vi "Dashboard Main.vi"() -> ()   [LabVIEW 2015]
uses:
  <vilib>/event_ctls.llb/eventvkey.ctl
  <vilib>/Utility/config.llb/NI_LVConfig.lvlib
  <vilib>/Utility/config.llb/Write Key (I32).vi
  <vilib>/Rock Robotics/WPI/Dashboard/WPI_DashboardLogging Global.vi
  <vilib>/Utility/config.llb/Write Key (String).vi
  <vilib>/Rock Robotics/Network Tables/NT Read Numeric Array.vi
  <vilib>/Utility/miscctls.llb/LVRowAndColumnTypeDef.ctl
panel:
  in  "TCP":refnum<k5>
  in  "Rec Mode":enum32{"Stop", "Record", "Playback"}(radio)
  in  "Vision":u16(ring) items=["Camera Off", "USB Camera SW", "USB Camera HW", "IP Camera"]
  out "Camera IP":string
  out "Image Message":string="Timeout in Camera Communications"
  in  "Dashboard Tab":T1(tab)
  in  "Select Auto":string(combo)
  out "NT Connection":bool
  in  "Camera Settings":T2={"Frame Rate"=30, "Compression"=30, "Size"=1} {"Frame Rate" scale=1.0..30.0; "Size" items=["640x480", "320x240", "160x120"]}
  out "MotorChart R":cluster{"Numeric":dbl, "Numeric":dbl}(graph)
  out "MotorChart L":T3(graph)
  out "MotorSliders R":cluster{"MotorSlide1":dbl, "MotorSlide2":dbl} {"MotorSlide2" scale=-1.0..1.0 scale format="%#_2e"; "MotorSlide1" scale=-1.0..1.0 scale format="%#_2e"}
  out "MotorSliders L":T4 {"MotorSlide4 2" scale=0.0..14.0 scale format="%#_2e"; "MotorSlide2" scale=-1.0..1.0 scale format="%#_2e"; "MotorSlide1" scale=-1.0..1.0 scale format="%#_2e"}
  out "Gyro":dbl(knob) scale=0.0..360.0
  out "JS1 Z":dbl(slide) scale=-1.0..1.0 scale format="%#_2e"
  out "JS1 Graph":cluster{"X":dbl, "Y":dbl}[](graph)
  out "JS1 Buttons":T5
  out "JS2 Z":dbl(slide) scale=-1.0..1.0 scale format="%#_2e"
  out "JS2 Graph":cluster{"X":dbl, "Y":dbl}[](graph)
  out "JS2 Buttons":T5
  out "Mode":T6(ring)=enum."Auto Disabled"
  in  "DB Camera Config":bool
  out "fps":dbl format="%#.1g"
  out "Mbps":dbl format="%#.1g"
  out "Mbps LED":bool
  in  "DB/String 9":string
  in  "DB/String 8":string
  in  "DB/String 7":string
  in  "DB/String 6":string
  in  "DB/String 5":string
  in  "DB/String 4":string
  in  "DB/String 3":string
  in  "DB/String 2":string
  in  "DB/String 1":string
  in  "DB/String 0":string
  in  "DB/Slider 0":dbl(slide) scale=0.0..5.0
  in  "DB/Slider 1":dbl(slide) scale=0.0..5.0
  in  "DB/Slider 2":dbl(slide) scale=0.0..5.0
  in  "DB/Slider 3":dbl(slide) scale=0.0..5.0
  out "DB/LED 3":bool
  out "DB/LED 2":bool
  out "DB/LED 1":bool
  out "DB/LED 0":bool
  in  "DB/Button 3":bool
  in  "DB/Button 2":bool
  in  "DB/Button 1":bool
  in  "DB/Button 0":bool caption="New Name"
  out "Aim":bool
  out "Shooter":bool
  out "Drive":bool
  in  "Strategty":i8 min=0 max=4
  in  "Test Slider":dbl(slide) scale=0.0..100.0 scale format="%#_3g"
  in  "On/Off":bool caption="Solenoid"
  in  "Test Name":u16(ring) items=["Select the test to run..."]
  in  "Test Tree":string(tree)
  in  "Motor":cluster{"Value":dbl, "Enable":bool} {"Value" scale=-1.0..1.0 scale format="%#_3g"}
  out "Progress":T7 {"Test Progress" scale=0.0..100.0}
  in  "Rev/Fwd":cluster{"Forward":bool, "Reverse":bool}
  in  "Test Ring":u16(ring) items=["Monochrome", "Color"]
  out "Cmd Status":string
  in  "Execute Command":bool
  in  "Command Params":string[][](table)
  in  "Command Selection":i32(listbox)
  in  "CheckList":i32(listbox)
  out "Tree":string(tree)
  out "Camera Image":T8(plugin-control)
  # "Left"
  # "Front"
  # "Right"
  # "Battery"
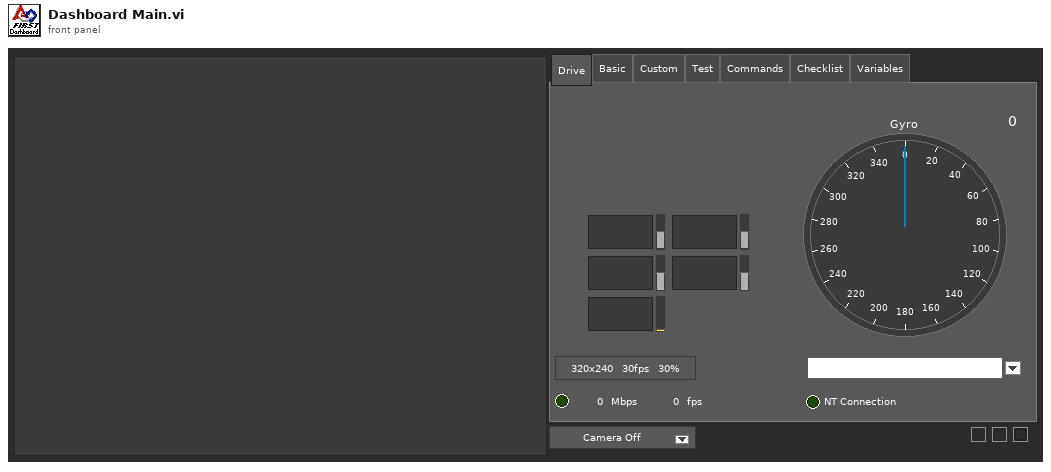
[diagram p1: front panel]
types:
  T1 = enum32{"Drive", "Basic", "Custom", "Test", "Commands", "Checklist", "Variables"}
  T2 = cluster{"Frame Rate":i32, "Compression":i32, "Size":u16}
  T3 = cluster{"Numeric":dbl, "Numeric":dbl, "Battery V":dbl}
  T4 = cluster{"MotorSlide1":dbl, "MotorSlide2":dbl, "MotorSlide4 2":dbl}
  T5 = cluster{bool, bool, bool, bool, bool, bool, bool, bool, bool, bool, bool, bool}
  T6 = enum8{"Tele-Op Disabled", "Tele-Op Enabled", "Auto Disabled", "Auto Enabled", "Test Disabled", "Test Enabled", "Disconnected", "No Code", "E-Stop"}
  T7 = cluster{"Test Progress":u8, "Test Progress Text":string}
  T8 = typedef "IMAQ Image.ctl" = refnum<image>
  T9 = cluster{"IDs":cluster{"RPC field ID":u16, "Unique ID":u16}, "String":string}
  T10 = enum32{"Drive", "Basic", "Custom", "Test", "Checklist", "Variables"}
  T11 = typedef "Image Type" = u32
  T12 = cluster{"Camera Image":refnum<vi>, "Dashboard Tab":refnum<vi>, void, "Vision":refnum<vi>, "Rec Mode":refnum<vi>, "Test Slider":refnum<vi>, "On/Off ":refnum<vi>, "Test Ring":refnum<vi>, "Rev/Fwd":refnum<vi>, "Test Name":refnum<vi>, "Motor":refnum<vi>, "Progress":refnum<vi>, "CheckList":refnum<vi>, "Tree":refnum<vi>, "Test Tree":refnum<vi>, "Command Params":refnum<vi>, "Command Selection":refnum<vi>, "Execute Command":refnum<vi>, "Cmd Status":refnum<vi>}
  T13 = cluster{"Error Strings":string, "Disable Counts":cluster{u16, u16}, "Rail Faults":cluster{u16, u16, u16}, "Robot IP":string, "DB Mode":u8, "Event Info":cluster{"Name":string, "Type":u8, "Number":u16, "Replay":u8}, "Camera Addr":string}
  T14 = cluster{"Storage":cluster{"Disk Free":u64, "RAM Block":u32, "RAM free":u32}, "CPU Utilization":cluster{"CPU % ISR":sgl, "CPU % Time Crit":sgl, "CPU % Timed Str":sgl, "CPU % High":sgl, "CPU % Above":sgl, "CPU % Normal":sgl, "CPU % Low":sgl}, "CAN":cluster{"% Bus Utilization":sgl, "Bus Off Cnt":u32, "TX_FIFO Full Cnt":u32, "Receive Error Cnt":u8, "Transmit Error Cnt":u8}, "HID":cluster{"HID Outputs":u32, "Rumble Low":u16, "Rumble High":u16}[]}
  T15 = cluster{"Status bits":cluster{"Test Mode":bool, "Autonomous":bool, "Enabled":bool, "Code Start":bool, "Brownout":bool, "Reserved 2":bool, "Reserved 3":bool, "E-Stop":bool}, "Code Trace":cluster{"Disabled":bool, "TeleOp":bool, "Auto":bool, "Test":bool}, "Controller Type":enum16{"unknown", "cRIO", "roboRio"}, "Code?":enum16{"unknown", "noCode", "code"}, "Battery V":dbl}
  T16 = cluster{"Control Bits":cluster{"TestMode":bool, "Autonomous":bool, "Enabled":bool, "FMS Present":bool, bool, bool, bool, "E-Stop":bool}, "Team Station ":u8, "Countdown":sgl, "Joystick Values":cluster{"Axes":dbl[], "Buttons":bool[], "POVs":i16[]}[]}
  T17 = cluster{"Axes":dbl[], "Buttons":bool[], "POVs":i16[]}[]
  T18 = cluster{"Axes":dbl[], "Buttons":bool[], "POVs":i16[]}
  T19 = cluster{"Buttons[0]":bool, "Buttons[1]":bool, "Buttons[2]":bool, "Buttons[3]":bool, "Buttons[4]":bool, "Buttons[5]":bool, "Buttons[6]":bool, "Buttons[7]":bool, "Buttons[8]":bool, "Buttons[9]":bool, "Buttons[10]":bool, "Buttons[11]":bool}
  T20 = typedef "NI_LVConfig.lvlib/Config Data RefNum.ctl" = refnum<k1>
  T21 = cluster{"Operation":enum16{"Update", "Clear"}, "Color Box":u32}[]
  T22 = typedef "eventvkey.ctl" = enum16{"ASCII", "Enter", "Return", "Shift", "Ctrl", "Alt", "Cmd", "Opt", "Caps", "NumLock", "Clear", "Break", "Up", "Down", "Left", "Right", "Insert", "Delete", "Home", "End", "PageUp", "PageDown", "Escape", "Help", "Pause", "ScrollLock", "F1", "F2", "F3", "F4", "F5", "F6", "F7", "F8", "F9", "F10", "F11", "F12", "F13", "F14", "F15", "F16", "F17", "F18", "F19", "F20", "F21", "F22", "F23", "F24", "Play", "VolumeUp", "VolumeDown", "Mute", "Two Byte Char"}
  T23 = cluster{"Image Size":bool, "Image Type":bool, "Pixel Value":bool, "ROI Information":bool, "Zoom Factor":bool}
  T24 = enum8{"Enabled", "Disabled", "Disabled and Grayed Out"}
  T25 = cluster{"Operation":enum16{"Update", "Clear"}, "Color Box":u32}
  T26 = typedef "LVRowAndColumnTypeDef.ctl" = cluster{"Row":i32, "Column":i32}
  T27 = cluster{"Shift":bool, "Ctrl":bool, "Alt":bool, "Cmd":bool, "Opt":bool}
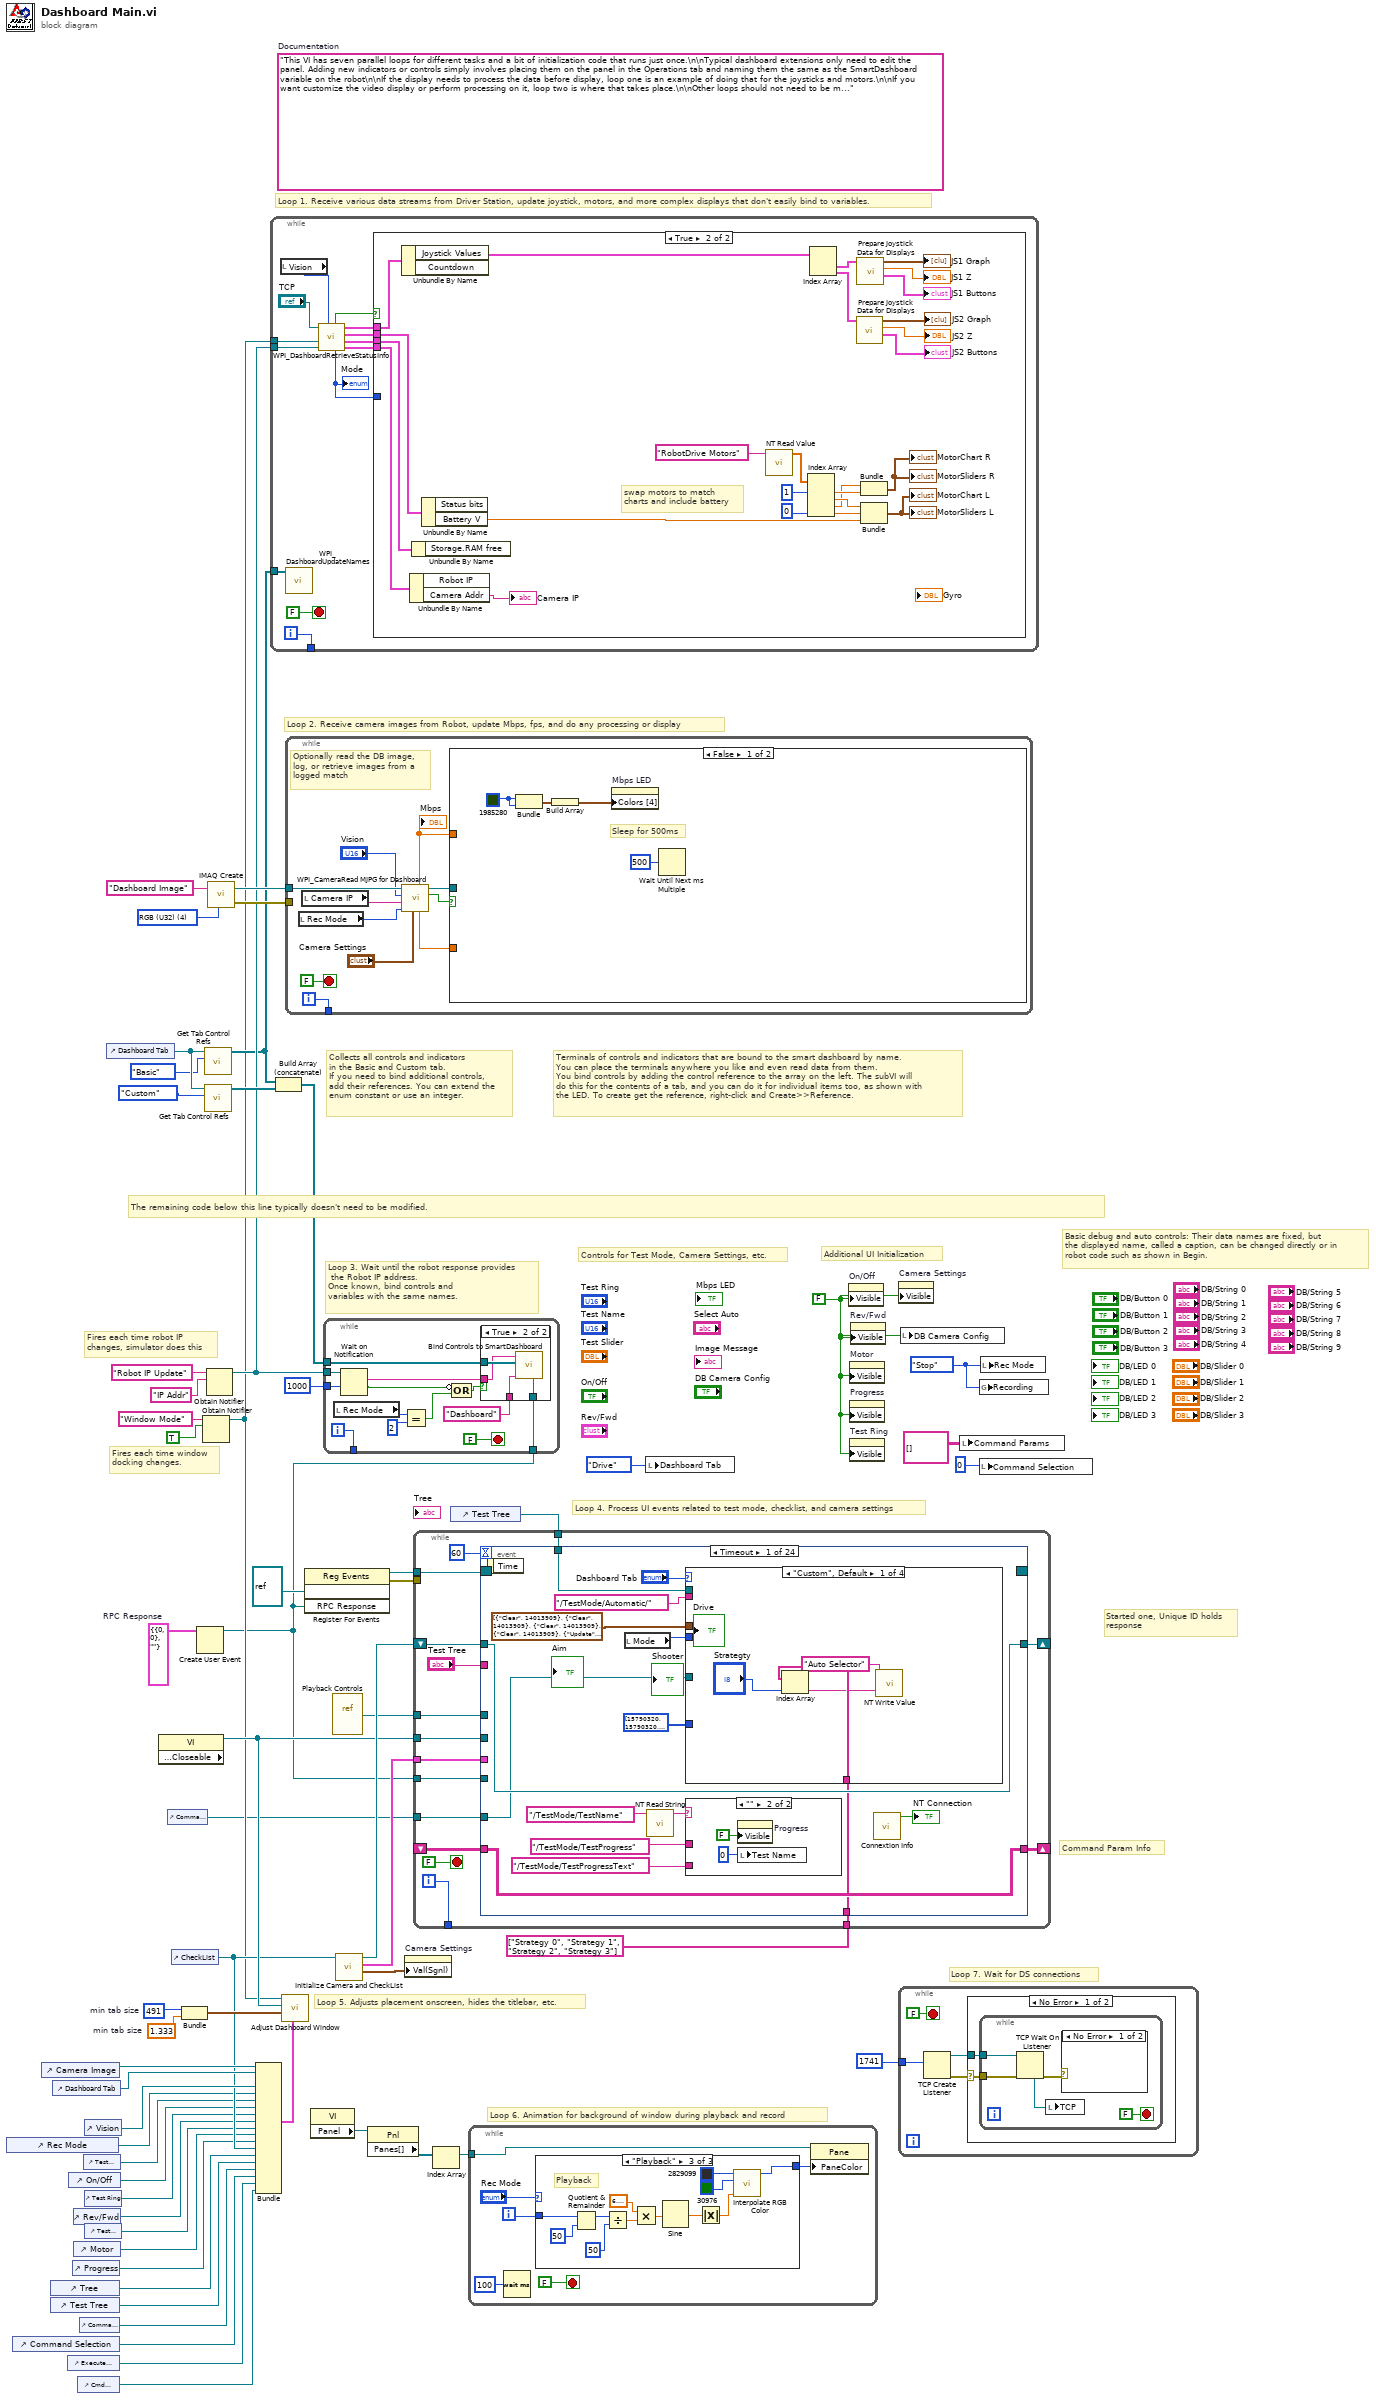
[diagram p0: block diagram]
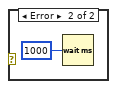
[diagram p2: hidden frame]
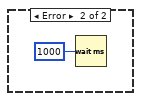
[diagram p3: hidden frame]
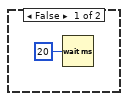
[diagram p4: hidden frame]
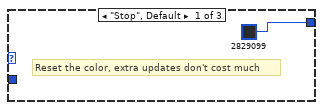
[diagram p5: hidden frame]
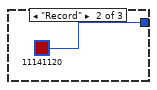
[diagram p6: hidden frame]
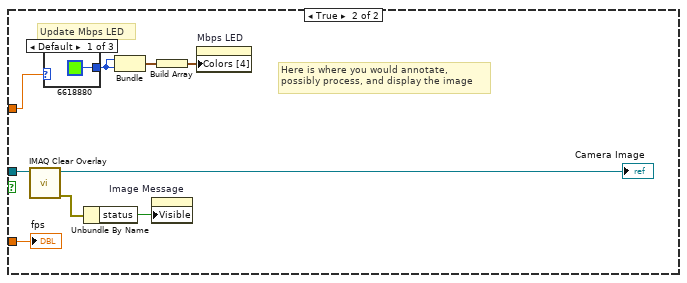
[diagram p8: hidden frame]
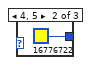
[diagram p9: hidden frame]
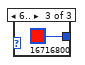
[diagram p10: hidden frame]
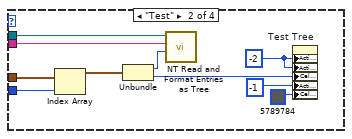
[diagram p11: hidden frame]
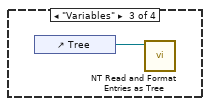
[diagram p12: hidden frame]
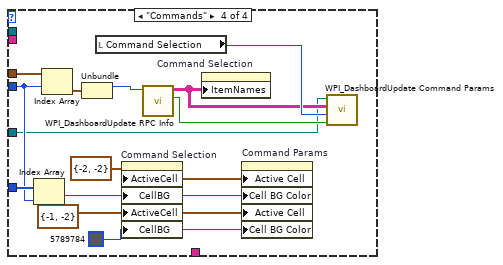
[diagram p13: hidden frame]
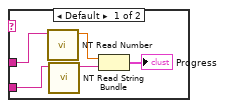
[diagram p14: hidden frame]
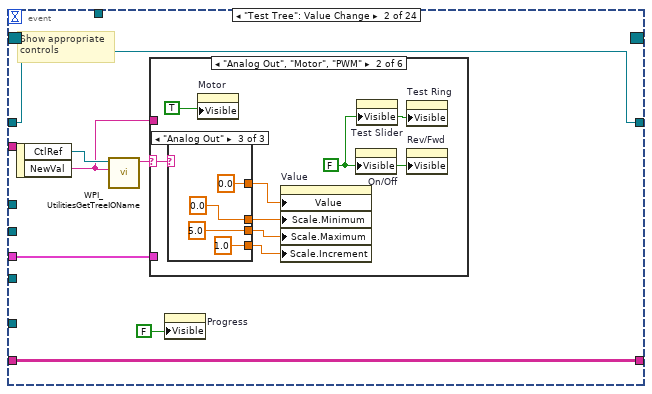
[diagram p15: hidden frame]
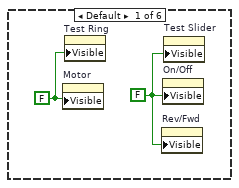
[diagram p16: hidden frame]
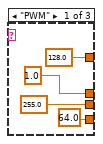
[diagram p17: hidden frame]
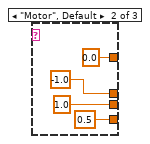
[diagram p18: hidden frame]
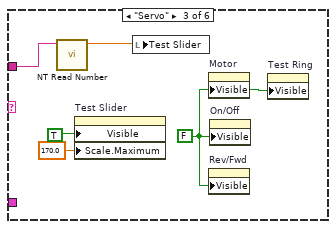
[diagram p19: hidden frame]
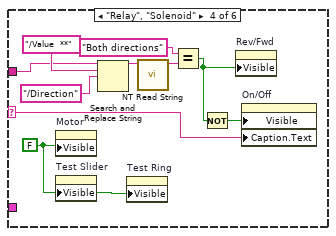
[diagram p20: hidden frame]
diagram:
  w8 = T9 {"IDs"={"RPC field ID"=0, "Unique ID"=0}, "String"=""}  # RPC Response
  w34 = 491  # min tab size
  w33 = 1.333  # min tab size
  w42 = enum32{"Stop", "Record", "Playback"}."Stop" ("Rec Mode")
  w16 = FALSE ("Visible")
  (unwired) "This VI has seven parallel loops for different tasks and a bit of initialization code that runs just once.\n\nTypical dashboard extensions only need to edit the panel. Adding new indicators or controls simply involves placing them on the panel in the Operations tab and naming them the same as the SmartDashboard variable on the robot\n\nIf the display needs to process the data before display, loop one is an example of doing that for the joysticks and motors.\n\nIf you want customize the video display or perform processing on it, loop two is where that takes place.\n\nOther loops should not need to be modified. They are pretty standard, and document the task they perform."  # Documentation
  w62 = T11 4 items=["Grayscale (U8)", "Grayscale (I16)", "Grayscale (SGL)", "Complex (CSG)", "RGB (U32)", "HSL (U32)", "RGB (U64)"] ("Image Type")
  # "Command Param Info"
  # "Started one, Unique ID holds\nresponse"
  # "Loop 7. Wait for DS connections"
  # "Basic debug and auto controls: Their data names are fixed, but\nthe displayed name, called a caption, can be changed directly or in\nrobot code such as shown in Begin."
  # "Controls for Test Mode, Camera Settings, etc."
  # "Additional UI Initialization"
  # "Loop 6. Animation for background of window during playback and record"
  # "Fires each time robot IP\nchanges, simulator does this"
  # "Fires each time window\ndocking changes."
  # "Collects all controls and indicators\nin the Basic and Custom tab.\nIf you need to bind additional controls,\nadd their references. You can extend the\nenum constant or use an integer."
  # "The remaining code below this line typically doesn't need to be modified."
  # "Loop 4. Process UI events related to test mode, checklist, and camera settings"
  # "Terminals of controls and indicators that are bound to the smart dashboard by name.\nYou can place the terminals anywhere you like and even read data from them.\nYou bind controls by adding the control reference to the array on the left. The subVI will\ndo this for the contents of a tab, and you can do it for individual items too, as shown with\nthe LED. To create get the reference, right-click and Create>>Reference."
  # "Loop 3. Wait until the robot response provides\n the Robot IP address.\nOnce known, bind controls and\nvariables with the same names."
  # "Loop 5. Adjusts placement onscreen, hides the titlebar, etc."
  # "Loop 1. Receive various data streams from Driver Station, update joystick, motors, and more complex displays that don't easily bind to variables."
  # "Loop 2. Receive camera images from Robot, update Mbps, fps, and do any processing or display"
  n1 = control-ref of="Rec Mode"() -> (w22:refnum<vi>)
  n2 = control-ref of="Command Selection"() -> (w7:refnum<vi>)
  n3 = control-ref of="Camera Image"() -> (w37:refnum<vi>)
  n4 = control-ref of="Tree"() -> (w26:refnum<vi>)
  n5 = control-ref of="Test Tree"() -> (w25:refnum<vi>)
  n6 = control-ref of="Dashboard Tab"() -> (w36:refnum<vi>)
  n7 = control-ref of="Execute Command"() -> (w9:refnum<vi>)
  n8 = control-ref of="On/Off"() -> (w20:refnum<vi>)
  n9 = control-ref of="Progress"() -> (w17:refnum<vi>)
  n10 = control-ref of="Rev/Fwd"() -> (w18:refnum<vi>)
  n11 = control-ref of="Motor"() -> (w23:refnum<vi>)
  n12 = control-ref of="Cmd Status"() -> (w3:refnum<vi>)
  n13 = control-ref of="Command Params"() -> (w10:refnum<vi>)
  n14 = control-ref of="Test Slider"() -> (w21:refnum<vi>)
  n15 = control-ref of="Vision"() -> (w35:refnum<vi>)
  n16 = control-ref of="Test Ring"() -> (w19:refnum<vi>)
  n17 = control-ref of="Test Name"() -> (w24:refnum<vi>)
  n18 = control-ref of="Dashboard Tab"() -> (w40:refnum<vi>)
  n19 = property class="VI" props=["Front Panel.Closeable"]() -> (reference out=w41:refnum<vi>)  [unwired: 2 in, 2 out]
  n20 = control-ref of="Command Params"() -> (w2:refnum<vi>)
  n21 = control-ref of="CheckList"() -> (w27:refnum<vi>)
  n22 = Bundle("min tab size"=w34, "min tab size"=w33) -> (w32:cluster{"min tab size":i32, "min tab size":dbl})  [unwired: 1 in]
  n23 = Create User Event(user event datatype=w8) -> (user event=w4:refnum<user-event>)  [unwired: 1 in, 1 out]
  n24 = Obtain Notifier(name (unnamed)="Window Mode", notification data type=TRUE) -> (notifier out=w13:refnum<notifier>)  [unwired: 2 in, 2 out]
  n25 = call <vilib>:"Get Tab Control Refs.vi"("Page Index"=T10."Basic" ("Dashboard Tab"), "TabControl in"=w40) -> ("ControlsOnPage"=w14:refnum<vi>[])  [unwired: 9 in]
  n26 = call <vilib>:"Get Tab Control Refs.vi"("Page Index"=T10."Custom" ("Dashboard Tab"), "TabControl in"=w40) -> ("ControlsOnPage"=w39:refnum<vi>[])  [unwired: 9 in]
  n27 = Obtain Notifier(name (unnamed)="Robot IP Update", notification data type="IP Addr" ("name (unnamed)")) -> (notifier out=w15:refnum<notifier>)  [unwired: 2 in, 2 out]
  n28 = call "IMAQ Create"("Image Name"="Dashboard Image", "Image Type"=w62) -> ("New Image"=w60:T8, "error out"=w59:errorcluster)  [unwired: 2 in, 1 out]
  n29 = Bundle("Camera Image"=w37, "Dashboard Tab"=w36, "Vision"=w35, "Rec Mode"=w22, "Test Slider"=w21, "On/Off"=w20, "Test Ring"=w19, "Rev/Fwd"=w18, "Test Name"=w24, "Motor"=w23, "Progress"=w17, "CheckList"=w27, "Tree"=w26, "Test Tree"=w25, "Command Params"=w10, "Command Selection"=w7, "Execute Command"=w9, "Cmd Status"=w3) -> (w28:T12, w31)  [unwired: 1 in]
  n30 = while {
    tunnel: [w74] -> _
    tunnel: w15 -> [w68]
    tunnel: w14 -> [w67]
    tunnel: w13 -> [w63]
    i -> [w74]
    stop <- FALSE stop-if-true
    n31 = local read "Vision"() -> (w65:u16)
    n32 = call <vilib>:"WPI_DashboardUpdateNames.vi"("Controls on Tab"=w67) -> ()  [unwired: 11 in]
    n33 = call <vilib>:"WPI_DashboardRetrieveStatusInfo.vi"("Vision"=w65, "Binding Refnum"=w68, "Window Mode Notifier"=w63, "TCP Cnx"="TCP") -> ("Power and Errors"=w69:T13, "Robot Metrics"=w72:T14, "Status Info"=w73:T15, "Control Info"=w70:T16, "Robot Mode"=w66:T6, "Process?"=w71:bool)  [unwired: 2 in]
    "Mode" <- w66
    n34 = case shown="True" w71 {
      tunnel: w73 -> [_ w101]
      tunnel: w72 -> [_ w100]
      tunnel: w70 -> [_ w99]
      tunnel: w69 -> [_ w98]
      tunnel: w66 -> [_ _]
      frame False {
        n35 = Wait (ms)(milliseconds to wait=u32 20) -> ()  [unwired: 1 out]
      }
      frame True {
        # "swap motors to match\ncharts and include battery"
        n36 = Unbundle By Name(w99) -> ("Joystick Values"=w88:T17)  [unwired: 1 out]
        n37 = Unbundle By Name(w98) -> ("Camera Addr"=→"Camera IP":string)  [unwired: 1 out]
        n38 = Unbundle By Name(w100) -> ()  [unwired: 1 out]
        n39 = Unbundle By Name(w101) -> ("Battery V"=w89:dbl)  [unwired: 1 out]
        n40 = call-poly <vilib>:"NT Read Value.vi"("Name"="RobotDrive Motors") -> ("Numeric Array"=w77:dbl[])  [unwired: 9 in, 1 out]
        n41 = Index Array(array=w77, index #1=1, index #4=0) -> (element #1=w93:dbl, element #2=w94:dbl, element #3=w92:dbl, element #4=w97:dbl)  [unwired: 2 in]
        n42 = Index Array(array=w88) -> (element #1=w87:T18, element #2=w82:T18)  [unwired: 2 in]
        n43 = call "Prepare Joystick Data for Displays.vi"("Joystick Values"=w82) -> ("Buttons"=→"JS2 Buttons":T19, "Z Axis"=→"JS2 Z":dbl, "Cartesian Data"=→"JS2 Graph":cluster{"X axis":dbl, "X axis":dbl}[])  [unwired: 8 in]
        n44 = call "Prepare Joystick Data for Displays.vi"("Joystick Values"=w87) -> ("Buttons"=→"JS1 Buttons":T19, "Z Axis"=→"JS1 Z":dbl, "Cartesian Data"=→"JS1 Graph":cluster{"X axis":dbl, "X axis":dbl}[])  [unwired: 8 in]
        n45 = Bundle("Numeric"=w92, "Numeric"=w93) -> (→"MotorChart R" →"MotorSliders R":cluster{"Numeric":dbl, "Numeric":dbl})  [unwired: 1 in]
        n46 = Bundle("Numeric"=w94, "Numeric"=w97, "Battery V"=w89) -> (→"MotorChart L" →"MotorSliders L":T3)  [unwired: 1 in]
      }
    }
  }
  n47 = Build Array (concatenate)(w14, w39) -> (w38:refnum<vi>[])
  n48 = call "Adjust Dashboard Window.vi"("Sizing Refnums"=w28, "Size Constraints"=w32, "VI"=w41, "WIn Mode"=w13) -> ()  [unwired: 8 in]
  n49 = while {
    tunnel: w60 -> [w110]
    tunnel: w59 -> [_]
    tunnel: [w111] -> _
    i -> [w111]
    stop <- FALSE stop-if-true
    # "Optionally read the DB image,\nlog, or retrieve images from a\nlogged match"
    n50 = local read "Rec Mode"() -> (w105:enum32{"Stop", "Record", "Playback"})
    n51 = local read "Camera IP"() -> (w103:string)
    n52 = call <vilib>:"WPI_CameraRead MJPG for Dashboard.vi"("Camera Settings"="Camera Settings", "Rec Mode"=w105, "Camera IP"=w103, "Camera Mode"="Vision", "Refnum in"=w110) -> ("Active"=w108:bool, "Refnum out"=w109:T8, "FPS"=w107:dbl, "Bandwidth (Mbps)"=w102:dbl)  [unwired: 3 in]
    "Mbps" <- w102
    n53 = case shown="False" w108 {
      tunnel: w109 -> [_ w120]
      tunnel: w102 -> [_ w119]
      tunnel: w107 -> [_ w117]
      frame False {
        w113 = u32 1985280 ("Color Box")
        # "Sleep for 500ms"
        n54 = Bundle("Color Box"=w113, "Color Box"=w113) -> (w115:cluster{"Color Box":u32, "Color Box":u32})  [unwired: 1 out]
        n55 = Build Array(w115) -> (w114:cluster{"Color Box":u32, "Color Box":u32}[])
        n56 = property on="Mbps LED" class="Bool (strict)"("Colors [4]"=w114) -> ()  [unwired: 2 in, 2 out]
        n57 = Wait Until Next ms Multiple(millisecond multiple=u32 500) -> ()  [unwired: 1 out]
      }
      frame True {
        # "Here is where you would annotate,\npossibly process, and display the image"
        # "Update Mbps LED"
        n58 = call "IMAQ Clear Overlay"("Image"=w120) -> ("error out"=w124:errorcluster, "Image Out"=→"Camera Image":T8)  [unwired: 2 in, 7 out]
        n59 = case shown="Default" w119 {
          tunnel: [u32 6618880 ("Color Box") u32 16776722 ("Color Box") u32 16716800 ("Color Box")] -> w121
          frame Default {
          }
          frame 4, 5 {
          }
          frame 6.. {
          }
        }
        n60 = Unbundle By Name(w124) -> ("status"=w125:bool)
        n61 = Bundle("Color Box"=w121, "Color Box"=w121) -> (w123:cluster{"Color Box":u32, "Color Box":u32})  [unwired: 1 out]
        n62 = property on="Image Message" class="Str"("Visible"=w125) -> ()  [unwired: 2 in, 2 out]
        n63 = Build Array(w123) -> (w122:cluster{"Color Box":u32, "Color Box":u32}[])
        n64 = property on="Mbps LED" class="Bool (strict)"("Colors [4]"=w122) -> ()  [unwired: 2 in, 2 out]
        "fps" <- w117
      }
    }
  }
  n65 = register-events(refnum<vi> refnum, w4) -> (reference out=w46:refnum<event-registration>, error out=w45:errorcluster)  [unwired: 2 in]
  n66 = property class="VI"() -> ("Panel"=w49:refnum<vi>)  [unwired: 2 in, 2 out]
  n67 = while {
    tunnel: w38 -> [w141]
    tunnel: w15 -> [w139]
    tunnel: [w137] -> _
    tunnel: u32 1000 ("milliseconds to wait") -> [w136]
    tunnel: w4 -> [w129]
    i -> [w137]
    stop <- FALSE stop-if-true
    n68 = local read "Rec Mode"() -> (w132:enum32{"Stop", "Record", "Playback"})
    n69 = Wait on Notification(notifier=w139, timeout in ms (-1)=w136) -> (notification=w138:string, timed out?=w134:bool)  [unwired: 2 in, 2 out]
    n70 = Equal?(x=w132, y=u16 2 ("Rec Mode")) -> (x = y?=w133:bool)
    n71 = Compound Arithmetic op=OR(invert w134, w133) -> (w135:bool)
    n72 = case shown="True" w135 {
      tunnel: w141 -> [_ w145]
      tunnel: w138 -> [_ w144]
      tunnel: "Dashboard" -> [_ w143]
      tunnel: w129 -> [_ w142]
      frame False {
      }
      frame True {
        n73 = call <vilib>:"Bind Controls to SmartDashboard.vi"("RPC ref"=w142, "Client Name"=w143, "Bound Control Refs"=w145, "Server IP Address"=w144) -> ()  [unwired: 8 in]
      }
    }
  }
  n74 = vi-ref "Playback Controls.vi"() -> (w47:refnum<vi>)
  n75 = call "Initialize Camera and CheckList.vi"("ListBox in"=w27) -> ("Cluster"=w53:cluster{"value":i32, "value":i32, "index":i32}, "Array"=w54:cluster{string[]}[], "File Refnum"=w52:T20)  [unwired: 8 in]
  n76 = property class="Pnl"(reference=w49) -> ("Panes[]"=w50:refnum<vi>[])  [unwired: 1 in, 2 out]
  n77 = property on="Camera Settings" class="Clust (strict)"("Val(Sgnl)"=w53) -> ()  [unwired: 2 in, 2 out]
  n78 = Index Array(array=w50) -> (element=w48:refnum<vi>)  [unwired: 1 in]
  n79 = control-ref of="Test Tree"() -> (w51:refnum<vi>)
  n80 = while {
    tunnel: w54 -> [w158]
    shift-right: [w157] -> _
    shift-left: w52 -> [w156]
    tunnel: [w155] -> _
    tunnel: w51 -> [w154]
    tunnel: w47 -> [w153]
    tunnel: w46 -> [w152]
    tunnel: w45 -> [_]
    tunnel: w41 -> [w151]
    tunnel: w4 -> [w150]
    tunnel: w2 -> [w149]
    shift-right: [w148] -> _
    shift-left: _ -> [w147]
    tunnel: string[] ["Strategy 0", "Strategy 1", "Strategy 2", "Strategy 3"] -> [w146]
    i -> [w155]
    stop <- FALSE stop-if-true
    n81 = event shown="[0] Timeout" {
      selector: w152 -> [_ _ _ _ _ _ _ _ _ _ _ _ _ _ _ _ _ _ _ _ _ _ _ _]
      dyn-events: [_ _ _ _ _ _ _ _ _ _ _ _ _ _ _ _ _ _ w472 _ _ _ _ _] -> _
      timeout: u32 60 ("milliseconds to wait") -> [_ _ _ _ _ _ _ _ _ _ _ _ _ _ _ _ _ _ _ _ _ _ _ _]
      tunnel: w154 -> [w172 _ _ _ _ _ _ _ _ _ _ _ _ _ _ _ _ _ _ _ _ _ _ _]
      tunnel: "Test Tree" -> [_ _ _ _ _ _ _ _ _ _ _ _ _ w435 w444 w447 w452 w461 _ _ _ _ _ _]
      tunnel: w158 -> [_ w214 _ _ _ _ _ _ _ _ _ w397 w428 _ _ _ _ _ _ _ _ _ _ _]
      tunnel: [w169 w213 w317 w323 w333 w337 w343 w355 w363 w369 w382 w396 w421 w434 w442 w446 w451 w460 w474 w490 w492 w500 w511 w516] -> w157
      tunnel: w156 -> [w169 w213 w317 w323 w333 w337 w343 w355 w363 w369 w382 w395 w421 w434 w442 w446 w451 w460 w474 w490 w492 w500 w511 w516]
      tunnel: w153 -> [_ _ _ _ _ _ _ _ _ _ _ _ _ _ _ _ _ _ w475 _ w495 _ _ _]
      tunnel: w151 -> [_ _ _ _ _ _ _ _ _ _ _ _ _ _ _ _ _ _ w470 _ _ _ _ _]
      tunnel: w150 -> [_ _ _ _ _ _ _ _ _ _ _ _ _ _ _ _ _ _ w466 _ _ _ _ _]
      tunnel: w149 -> [w164 _ _ _ _ _ w341 _ _ _ _ _ _ _ _ _ _ _ _ _ _ _ _ _]
      tunnel: [w163 w212 w316 w322 w332 w338 w339 w349 w360 w368 w381 w394 w420 w433 w441 w445 w450 w459 w465 w488 w491 w496 w504 w517] -> w148
      tunnel: w147 -> [w163 w212 w316 w322 w332 w338 w339 _ _ w368 w381 w394 w420 w433 w441 w445 w450 w459 w465 w488 w491 w496 w504 w517]
      tunnel: w146 -> [w162 _ _ _ _ _ _ _ _ _ _ _ _ _ _ _ _ _ _ _ _ _ _ _]
      event Timeout {
        n82 = event-data() -> ()  [unwired: 1 in, 1 out]
        n83 = local read "Mode"() -> (w166:T6)
        n84 = call <vilib>:"NT Read String.vi"("Name"="/TestMode/TestName") -> ("String"=w175:string)  [unwired: 9 in, 1 out]
        n85 = case shown="\"Custom\", Default" "Dashboard Tab" {
          tunnel: w172 -> [_ w190 _ _]
          tunnel: "/TestMode/Automatic/" ("Name Pattern") -> [_ w189 _ _]
          tunnel: T21 [{"Operation"=enum."Clear", "Color Box"=14013909}, {"Operation"=enum."Clear", "Color Box"=14013909}, {"Operation"=enum."Clear", "Color Box"=14013909}, {"Operation"=enum."Clear", "Color Box"=14013909}, {"Operation"=enum."Update", "Color Box"=14013909}, {"Operation"=enum."Update", "Color Box"=16777215}, {"Operation"=enum."Clear", "Color Box"=14013909}, {"Operation"=enum."Clear", "Color Box"=14013909}, {"Operation"=enum."Clear", "Color Box"=14013909}] -> [_ w182 _ w199]
          tunnel: w166 -> [_ w181 _ w198]
          tunnel: u32[] [15790320, 15790320, 15790320, 15790320, 16777215, 16777215, 15790320, 15790320, 15790320] -> [_ _ _ w204]
          tunnel: w164 -> [_ _ _ w192]
          tunnel: w162 -> [w179 _ _ _]
          frame "Custom", Default {
            n86 = Index Array(array=w179, index="Strategty") -> (element=w178:string)
            n87 = call-poly <vilib>:"NT Write Value.vi"("String"=w178, "Name"="Auto Selector") -> ()  [unwired: 9 in, 1 out]
          }
          frame "Test" {
            w188 = -2 ("Active Item:Row Number")
            n88 = Index Array(array=w182, index=w181) -> (element=w183:T25)
            n89 = Unbundle(w183) -> ("Operation"=w184:enum16{"Update", "Clear"}, "Color Box"=w185:u32)
            n90 = call <vilib>:"NT Read and Format Entries as Tree.vi"("Operation"=w184, "Name Pattern"=w189, "Tree Refnum"=w190) -> ()  [unwired: 7 in, 2 out]
            n91 = property on="Test Tree" class="Tree (strict)"("Active Item Row Number"=w188, "ActiveColNum"=w188, "CellBG"=w185, "Active Item Row Number"=-1 ("Active Item:Row Number"), "CellBG"=u32 5789784 ("Color Box")) -> ()  [unwired: 2 in, 2 out]
          }
          frame "Variables" {
            n92 = control-ref of="Tree"() -> (w191:refnum<vi>)
            n93 = call <vilib>:"NT Read and Format Entries as Tree.vi"("Tree Refnum"=w191) -> ()  [unwired: 9 in, 2 out]
          }
          frame "Commands" {
            w200 = u32 5789784 ("Color Box")
            w201 = T26 {"Row"=-1, "Column"=-2} ("Active Cell:Active Cell")
            w203 = T26 {"Row"=-2, "Column"=-2} ("Active Cell:Active Cell")
            n94 = Index Array(array=w204, index=w198) -> (element=w202:u32)
            n95 = Index Array(array=w199, index=w198) -> (element=w197:T25)
            n96 = Unbundle(w197) -> ("Operation"=w196:enum16{"Update", "Clear"})  [unwired: 1 out]
            n97 = local read "Command Selection"() -> (w195:i32)
            n98 = property on="Command Selection" class="MCListbox (strict)"("ActiveCell"=w203, "CellBG"=w202, "ActiveCell"=w201, "CellBG"=w200) -> ()  [unwired: 2 in, 2 out]
            n99 = call <vilib>:"WPI_DashboardUpdate RPC Info.vi"("Operation"=w196) -> ("update"=w194:bool, "commands"=w193:string[][])  [unwired: 9 in]
            n100 = property on="Command Selection" class="MCListbox (strict)"("ItemNames"=w193) -> ()  [unwired: 2 in, 2 out]
            n101 = property on="Command Params" class="Tbl (strict)"("Active Cell"=w203, "Cell BG Color"=w202, "Active Cell"=w201, "Cell BG Color"=w200) -> ()  [unwired: 2 in, 2 out]
            n102 = call <vilib>:"WPI_DashboardUpdate Command Params.vi"("Update"=w194, "NewVal"=w195, "Commands"=w193, "Param Tbl"=w192) -> ()  [unwired: 7 in, 1 out]
          }
        }
        n103 = case shown="\"\"" w175 {
          tunnel: "/TestMode/TestProgress" ("Name") -> [w206 _]
          tunnel: "/TestMode/TestProgressText" ("Name") -> [w205 _]
          frame Default {
            n104 = call <vilib>:"NT Read Number.vi"("Name"=w206) -> ("Numeric"=w207:dbl)  [unwired: 9 in, 1 out]
            n105 = call <vilib>:"NT Read String.vi"("Name"=w205) -> ("String"=w208:string)  [unwired: 9 in, 1 out]
            n106 = Bundle("Numeric"=w207, "String"=w208) -> (→"Progress":cluster{"Numeric":dbl, "String":string})  [unwired: 1 in]
          }
          frame "" {
            n107 = property on="Progress" class="Clust (strict)"("Visible"=FALSE) -> ()  [unwired: 2 in, 2 out]
            n108 = local write "Test Name"(u16 0) -> ()
          }
        }
        n109 = call <vilib>:"Connextion Info.vi"() -> ("Connected"=→"NT Connection":bool)  [unwired: 10 in, 1 out]
      }
      event "Test Tree": Value Change {
        # "Show appropriate\ncontrols"
        n110 = event-data() -> ("CtlRef"=w217:refnum<vi>, "NewVal"=w215:string)  [unwired: 1 in]
        n111 = call <vilib>:"WPI_UtilitiesGetTreeIOName.vi"("NewVal"=w215, "TreeControl in"=w217) -> ("I/O Name"=w218:string)  [unwired: 9 in]
        n112 = case shown="\"Analog Out\", \"Motor\", \"PWM\"" w218 {
          selector: w218 -> [_ w225 _ w247 w256 _]
          tunnel: w215 -> [_ _ w244 w246 _ w263]
          tunnel: w214 -> [_ _ _ _ _ w262]
          frame Default {
            w220 = FALSE ("Visible")
            w219 = FALSE ("Visible")
            n113 = property on="Motor" class="Clust (strict)"("Visible"=w219) -> ()  [unwired: 2 in, 2 out]
            n114 = property on="Test Ring" class="Ring (strict)"("Visible"=w219) -> ()  [unwired: 2 in, 2 out]
            n115 = property on="Rev/Fwd" class="Clust (strict)"("Visible"=w220) -> ()  [unwired: 2 in, 2 out]
            n116 = property on="On/Off" class="Bool (strict)"("Visible"=w220) -> ()  [unwired: 2 in, 2 out]
            n117 = property on="Test Slider" class="Slide (strict)"("Visible"=w220) -> ()  [unwired: 2 in, 2 out]
          }
          frame "Analog Out", "Motor", "PWM" {
            w226 = FALSE ("Visible")
            n118 = case shown="\"Analog Out\"" w225 {
              tunnel: [1.0 ("Value") -1.0 ("Value") 0.0 ("Value")] -> w224
              tunnel: [255.0 ("Value") 1.0 ("Value") 5.0 ("Value")] -> w223
              tunnel: [128.0 ("Value") 0.0 ("Value") 0.0 ("Value")] -> w222
              tunnel: [64.0 ("Value") 0.5 ("Value") 1.0 ("Value")] -> w221
              frame "PWM" {
              }
              frame "Motor", Default {
              }
              frame "Analog Out" {
              }
            }
            n119 = property on="Motor" class="Clust (strict)"("Visible"=TRUE) -> ()  [unwired: 2 in, 2 out]
            n120 = property on="Value" class="Slide (strict)"("Value"=w222, "Scale.Minimum"=w224, "Scale.Maximum"=w223, "Scale.Increment"=w221) -> ()  [unwired: 2 in, 2 out]
            n121 = property on="On/Off" class="Bool (strict)"("Visible"=w226) -> ()  [unwired: 2 in, 2 out]
            n122 = property on="Test Slider" class="Slide (strict)"("Visible"=w226) -> ()  [unwired: 2 in, 2 out]
            n123 = property on="Test Ring" class="Ring (strict)"("Visible"=w226) -> ()  [unwired: 2 in, 2 out]
            n124 = property on="Rev/Fwd" class="Clust (strict)"("Visible"=w226) -> ()  [unwired: 2 in, 2 out]
          }
          frame "Servo" {
            w242 = FALSE ("Visible")
            n125 = call <vilib>:"NT Read Number.vi"("Name"=w244) -> ("Numeric"=w243:dbl)  [unwired: 9 in, 1 out]
            n126 = property on="Test Slider" class="Slide (strict)"("Visible"=TRUE, "Scale.Maximum"=170.0 ("Scale.Range:Maximum")) -> ()  [unwired: 2 in, 2 out]
            n127 = local write "Test Slider"(w243) -> ()
            n128 = property on="Motor" class="Clust (strict)"("Visible"=w242) -> ()  [unwired: 2 in, 2 out]
            n129 = property on="Rev/Fwd" class="Clust (strict)"("Visible"=w242) -> ()  [unwired: 2 in, 2 out]
            n130 = property on="On/Off" class="Bool (strict)"("Visible"=w242) -> ()  [unwired: 2 in, 2 out]
            n131 = property on="Test Ring" class="Ring (strict)"("Visible"=w242) -> ()  [unwired: 2 in, 2 out]
          }
          frame "Relay", "Solenoid" {
            w245 = FALSE ("Visible")
            n132 = property on="Motor" class="Clust (strict)"("Visible"=w245) -> ()  [unwired: 2 in, 2 out]
            n133 = property on="Test Slider" class="Slide (strict)"("Visible"=w245) -> ()  [unwired: 2 in, 2 out]
            n134 = Search and Replace String(input string=w246, search string="/Value  **", replace string="/Direction") -> (result string=w252:string)  [unwired: 5 in, 3 out]
            n135 = property on="Test Ring" class="Ring (strict)"("Visible"=w245) -> ()  [unwired: 2 in, 2 out]
            n136 = call <vilib>:"NT Read String.vi"("Name"=w252) -> ("String"=w250:string)  [unwired: 9 in, 1 out]
            n137 = Equal?(x="Both directions", y=w250) -> (x = y?=w248:bool)
            n138 = Not(x=w248) -> (.not. x?=w249:bool)
            n139 = property on="Rev/Fwd" class="Clust (strict)"("Visible"=w248) -> ()  [unwired: 2 in, 2 out]
            n140 = property on="On/Off" class="Bool (strict)"("Visible"=w249, "Caption.Text"=w247) -> ()  [unwired: 2 in, 2 out]
          }
          frame "Compressor", "Digital Out" {
            w255 = FALSE ("Visible")
            # "Get direction and finish"
            n141 = property on="Motor" class="Clust (strict)"("Visible"=w255) -> ()  [unwired: 2 in, 2 out]
            n142 = property on="Test Slider" class="Slide (strict)"("Visible"=w255) -> ()  [unwired: 2 in, 2 out]
            n143 = property on="Test Ring" class="Ring (strict)"("Visible"=w255) -> ()  [unwired: 2 in, 2 out]
            n144 = property on="On/Off" class="Bool (strict)"("Visible"=TRUE, "Caption.Text"=w256) -> ()  [unwired: 2 in, 2 out]
            n145 = property on="Rev/Fwd" class="Clust (strict)"("Visible"=FALSE) -> ()  [unwired: 2 in, 2 out]
          }
          frame "Camera" {
            n146 = call <vilib>:"Get Last Path Segment.vi"("String in"=w263) -> ("String out"=w264:string)  [unwired: 10 in]
            n147 = property on="On/Off" class="Bool (strict)"("Visible"=FALSE) -> ()  [unwired: 2 in, 2 out]
            n148 = property on="Motor" class="Clust (strict)"("Visible"=FALSE) -> ()  [unwired: 2 in, 2 out]
            n149 = property on="Rev/Fwd" class="Clust (strict)"("Visible"=FALSE) -> ()  [unwired: 2 in, 2 out]
            n150 = case shown="\"White Balance  **\"" w264 {
              tunnel: w263 -> [w270 w279 w288 w297 w306 _ w312]
              tunnel: w262 -> [w268 w276 w285 w294 w303 _ _]
              frame "Size  **" {
                n151 = Index Array(array=w268) -> (element=w267:cluster{string[]})  [unwired: 1 in]
                n152 = call <vilib>:"NT Read String.vi"("Name"=w270) -> ("String"=w269:string)  [unwired: 9 in, 1 out]
                n153 = Unbundle(w267) -> (w265:string[])
                n154 = Match First String(2:w265, 3:w269) -> (0:w266:i32)  [unwired: 1 out]
                n155 = property on="Test Ring" class="Ring (strict)"("Value"=w266, "Strings []"=w265) -> ()  [unwired: 2 in, 2 out]
                n156 = property on="Test Ring" class="Ring (strict)"("Visible"=TRUE) -> ()  [unwired: 2 in, 2 out]
                n157 = property on="Test Slider" class="Slide (strict)"("Visible"=FALSE) -> ()  [unwired: 2 in, 2 out]
              }
              frame "White Balance  **" {
                n158 = Index Array(array=w276, index=1) -> (element=w277:cluster{string[]})
                n159 = call <vilib>:"NT Read String.vi"("Name"=w279) -> ("String"=w278:string)  [unwired: 9 in, 1 out]
                n160 = Unbundle(w277) -> (w274:string[])
                n161 = Match First String(2:w274, 3:w278) -> (0:w273:i32)  [unwired: 1 out]
                n162 = property on="Test Ring" class="Ring (strict)"("Value"=w273, "Strings []"=w274) -> ()  [unwired: 2 in, 2 out]
                n163 = property on="Test Ring" class="Ring (strict)"("Visible"=TRUE) -> ()  [unwired: 2 in, 2 out]
                n164 = property on="Test Slider" class="Slide (strict)"("Visible"=FALSE) -> ()  [unwired: 2 in, 2 out]
              }
              frame "Exposure  **" {
                n165 = Index Array(array=w285, index=2) -> (element=w286:cluster{string[]})
                n166 = call <vilib>:"NT Read String.vi"("Name"=w288) -> ("String"=w287:string)  [unwired: 9 in, 1 out]
                n167 = Unbundle(w286) -> (w282:string[])
                n168 = Match First String(2:w282, 3:w287) -> (0:w283:i32)  [unwired: 1 out]
                n169 = property on="Test Ring" class="Ring (strict)"("Value"=w283, "Strings []"=w282) -> ()  [unwired: 2 in, 2 out]
                n170 = property on="Test Ring" class="Ring (strict)"("Visible"=TRUE) -> ()  [unwired: 2 in, 2 out]
                n171 = property on="Test Slider" class="Slide (strict)"("Visible"=FALSE) -> ()  [unwired: 2 in, 2 out]
              }
              frame "Exposure Priority  **" {
                n172 = Index Array(array=w294, index=3) -> (element=w295:cluster{string[]})
                n173 = call <vilib>:"NT Read String.vi"("Name"=w297) -> ("String"=w296:string)  [unwired: 9 in, 1 out]
                n174 = Unbundle(w295) -> (w291:string[])
                n175 = Match First String(2:w291, 3:w296) -> (0:w292:i32)  [unwired: 1 out]
                n176 = property on="Test Ring" class="Ring (strict)"("Value"=w292, "Strings []"=w291) -> ()  [unwired: 2 in, 2 out]
                n177 = property on="Test Ring" class="Ring (strict)"("Visible"=TRUE) -> ()  [unwired: 2 in, 2 out]
                n178 = property on="Test Slider" class="Slide (strict)"("Visible"=FALSE) -> ()  [unwired: 2 in, 2 out]
              }
              frame "Color Enable  **" {
                n179 = Index Array(array=w303, index=4) -> (element=w304:cluster{string[]})
                n180 = call <vilib>:"NT Read String.vi"("Name"=w306) -> ("String"=w305:string)  [unwired: 9 in, 1 out]
                n181 = Unbundle(w304) -> (w300:string[])
                n182 = Match First String(2:w300, 3:w305) -> (0:w301:i32)  [unwired: 1 out]
                n183 = property on="Test Ring" class="Ring (strict)"("Value"=w301, "Strings []"=w300) -> ()  [unwired: 2 in, 2 out]
                n184 = property on="Test Ring" class="Ring (strict)"("Visible"=TRUE) -> ()  [unwired: 2 in, 2 out]
                n185 = property on="Test Slider" class="Slide (strict)"("Visible"=FALSE) -> ()  [unwired: 2 in, 2 out]
              }
              frame Default {
                n186 = property on="Test Ring" class="Ring (strict)"("Visible"=FALSE) -> ()  [unwired: 2 in, 2 out]
                n187 = property on="Test Slider" class="Slide (strict)"("Visible"=FALSE) -> ()  [unwired: 2 in, 2 out]
              }
              frame "Brightness  **", "Color Level  **", "Compression  **", "FPS  **", "Sharpness  **" {
                n188 = call <vilib>:"NT Read Number.vi"("Name"=w312) -> ("Numeric"=w311:dbl)  [unwired: 9 in, 1 out]
                n189 = local write "Test Slider"(w311) -> ()
                n190 = property on="Test Slider" class="Slide (strict)"("Visible"=TRUE, "Scale.Maximum"=100.0 ("Scale.Range:Maximum")) -> ()  [unwired: 2 in, 2 out]
                n191 = property on="Test Ring" class="Ring (strict)"("Visible"=FALSE) -> ()  [unwired: 2 in, 2 out]
              }
            }
          }
        }
        n192 = property on="Progress" class="Clust (strict)"("Visible"=FALSE) -> ()  [unwired: 2 in, 2 out]
      }
      event "Test Name": Mouse Enter {
        # "Populate the ring with the list of tests"
        n193 = event-data() -> ()  [unwired: 1 in, 1 out]
        n194 = call <vilib>:"NT Read String Array.vi"("Name"="/TestMode/TestList") -> ("String Array"=w321:string[])  [unwired: 9 in, 1 out]
        n195 = Build Array (concatenate)("Select the test to run...", w321) -> (w320:string[])
        n196 = property on="Test Name" class="Ring (strict)"("Strings []"=w320) -> ()  [unwired: 2 in, 2 out]
      }
      event "Test Name": Value Change {
        w324 = FALSE ("Visible")
        # "Tell the robot the test name to run"
        n197 = event-data() -> ("NewVal"=w328:u16)  [unwired: 1 in]
        n198 = property on="Test Name" class="Ring (strict)"() -> ("Strings []"=w329:string[])  [unwired: 2 in, 2 out]
        n199 = local write "Progress"(T7 {"Test Progress"=0, "Test Progress Text"=""} ("Progress")) -> ()
        n200 = Index Array(array=w329, index=w328) -> (element=w327:string)
        n201 = call <vilib>:"NT Write String.vi"("String"=w327, "Name"="/TestMode/TestName") -> ()  [unwired: 9 in, 1 out]
        n202 = property on="Progress" class="Clust (strict)"("Visible"=TRUE) -> ()  [unwired: 2 in, 2 out]
        n203 = property on="Motor" class="Clust (strict)"("Visible"=w324) -> ()  [unwired: 2 in, 2 out]
        n204 = property on="Test Slider" class="Slide (strict)"("Visible"=w324) -> ()  [unwired: 2 in, 2 out]
        n205 = property on="On/Off" class="Bool (strict)"("Visible"=w324) -> ()  [unwired: 2 in, 2 out]
        n206 = property on="Rev/Fwd" class="Clust (strict)"("Visible"=w324) -> ()  [unwired: 2 in, 2 out]
        n207 = property on="Test Ring" class="Ring (strict)"("Visible"=w324) -> ()  [unwired: 2 in, 2 out]
      }
      event "Select Auto": Mouse Enter {
        # "Populate the combo box with the list of autonomous options"
        n208 = event-data() -> ()  [unwired: 1 in, 1 out]
        n209 = call <vilib>:"NT Read String Array.vi"("Name"="Auto List") -> ("String Array"=w331:string[])  [unwired: 9 in, 1 out]
        n210 = property on="Select Auto" class="CmbBox"("Strings[]"=w331) -> ()  [unwired: 2 in, 2 out]
      }
      event "Select Auto": Value Change {
        # "User modified the Auto Selection. Write to NT variable so robot knows."
        n211 = event-data() -> ("NewVal"=w335:string)  [unwired: 1 in]
        n212 = call <vilib>:"NT Write String.vi"("String"=w335, "Name"="Auto Selector") -> ()  [unwired: 9 in, 1 out]
      }
      event "Command Selection": Value Change {
        # "Get the params and show in table"
        n213 = event-data() -> ("NewVal"=w342:i32)  [unwired: 1 in]
        n214 = property on="Command Selection" class="MCListbox (strict)"() -> ("ItemNames"=w340:string[][])  [unwired: 2 in, 2 out]
        n215 = call <vilib>:"WPI_DashboardUpdate Command Params.vi"("NewVal"=w342, "Commands"=w340, "Param Tbl"=w341) -> ()  [unwired: 8 in, 1 out]
      }
      event "Execute Command": Value Change {
        # "Started one, Unique ID holds\nresponse"
        n216 = event-data() -> ()  [unwired: 1 in, 1 out]
        n217 = property on="Command Selection" class="MCListbox (strict)"() -> ("ItemNames"=w354:string[][])  [unwired: 2 in, 2 out]
        n218 = Index Array(array=w354, index (row)="Command Selection", index (col)=0) -> (element=w352:string)
        n219 = call <vilib>:"Invoke Commands.vi"("Command Params"="Command Params", "Function Name"=w352) -> ("Params"=w348:u8, "Started"=w347:bool)  [unwired: 7 in, 1 out]
        n220 = Array Subset(array="Command Params", length (row)=w348) -> (w349:string[][])  [unwired: 3 in]
        n221 = Select(t="Executing" ("Cmd Status"), s=w347, f="" ("Cmd Status")) -> (s? t:f=→"Cmd Status":string)
      }
      event "Command Selection": Double Click {
        n222 = event-data() -> ("Row"=w364:i32)  [unwired: 1 in]
        n223 = property on="Command Selection" class="MCListbox (strict)"() -> ("ItemNames"=w367:string[][])  [unwired: 2 in, 2 out]
        n224 = local read "Command Params"() -> (w362:string[][])
        n225 = Index Array(array=w367, index (row)=w364, index (col)=0) -> (element=w365:string)
        n226 = call <vilib>:"Invoke Commands.vi"("Command Params"=w362, "Function Name"=w365) -> ("Params"=w361:u8, "Started"=w356:bool)  [unwired: 7 in, 1 out]
        n227 = Array Subset(array=w362, length (row)=w361) -> (w360:string[][])  [unwired: 3 in]
        n228 = Select(t="Executing" ("Cmd Status"), s=w356, f="" ("Cmd Status")) -> (s? t:f=w357:string)
        n229 = local write "Cmd Status"(w357) -> ()
      }
      event "CheckList": Double Click {
        # "Shift clears all"
        # "Update symbols on the listbox"
        n230 = event-data() -> ("PlatMods.Shift"=w370:bool, "Row"=w372:i32)  [unwired: 1 in]
        n231 = case shown="True" w370 {
          tunnel: w372 -> [w376 _]
          tunnel: 1 -> [w375 _]
          frame False {
            n232 = property on="CheckList" class="LstBox (strict)"() -> ("Item Symbols"=w374:i32[])  [unwired: 2 in, 2 out]
            n233 = Replace Array Subset(array=w374, new element=w375, index=w376) -> (w373:i32[])
            n234 = property on="CheckList" class="LstBox (strict)"("Item Symbols"=w373) -> ()  [unwired: 2 in, 2 out]
          }
          frame True {
            w377 = 0 ("Top Row")
            n235 = property on="CheckList" class="LstBox (strict)"() -> ("Number of Rows"=w379:u32)  [unwired: 2 in, 2 out]
            n236 = Initialize Array(0, w379) -> (w378:i32[])
            n237 = property on="CheckList" class="LstBox (strict)"("Top Row"=w377, "Value"=w377, "Item Symbols"=w378) -> ()  [unwired: 2 in, 2 out]
          }
        }
      }
      event "CheckList": Key Down {
        # "Update symbols on the listbox\nLeft and right keys check and uncheck"
        n238 = event-data() -> ("VKey"=w384:T22)  [unwired: 1 in]
        n239 = case shown="\"Left\", \"Right\"" w384 {
          selector: w384 -> [w389 _]
          tunnel: eventvkey."Left" ("VKey") -> [w387 _]
          frame "Left", "Right" {
            n240 = Equal?(x=w387, y=w389) -> (x = y?=w388:bool)
            n241 = Select(t=0, s=w388, f=1) -> (s? t:f=w390:i32)
            n242 = property on="CheckList" class="LstBox (strict)"() -> ("Item Symbols"=w393:i32[])  [unwired: 2 in, 2 out]
            n243 = Replace Array Subset(array=w393, new element=w390, index="CheckList") -> (w392:i32[])
            n244 = property on="CheckList" class="LstBox (strict)"("Item Symbols"=w392) -> ()  [unwired: 2 in, 2 out]
          }
          frame Default {
          }
        }
      }
      event "DB Camera Config": Value Change {
        # "Show or hide the cluster of controls, store in ini file"
        n245 = event-data() -> ("NewVal"=w398:bool)  [unwired: 1 in]
        n246 = case shown="False" w398 {
          tunnel: w397 -> [w407 _]
          tunnel: [w400 w418] -> w396
          tunnel: w395 -> [w399 w418]
          frame False {
            w414 = "Camera"
            w417 = FALSE ("Visible")
            n247 = local read "Camera Settings"() -> (w406:T2)
            n248 = Index Array(array=w407) -> (element=w410:cluster{string[]})  [unwired: 1 in]
            n249 = Unbundle(w406) -> ("Frame Rate"=w405:i32, "Compression"=w404:i32, "Size"=w408:u16)
            n250 = Unbundle(w410) -> (w409:string[])
            n251 = Index Array(array=w409, index=w408) -> (element=w403:string)
            n252 = call-poly <vilib>:"Write Key.vi"("section"=w414, "value"=w403, "key"="Size", "refnum"=w399) -> ("refnum out"=w416:T20)  [unwired: 2 in, 5 out]
            n253 = call-poly <vilib>:"Write Key.vi"("section"=w414, "value"=w405, "key"="FrameRate", "refnum"=w416) -> ("refnum out"=w415:T20)  [unwired: 1 in, 6 out]
            n254 = property on="Camera Settings" class="Clust (strict)"("Visible"=w417) -> ()  [unwired: 2 in, 2 out]
            n255 = local write "DB Camera Config"(w417) -> ()
            n256 = call-poly <vilib>:"Write Key.vi"("section"=w414, "value"=w404, "key"="Compression", "refnum"=w415) -> ("refnum out"=w401:T20)  [unwired: 1 in, 6 out]
            n257 = call <vilib>:"Close Config Data.vi"("refnum"=w401) -> ("file path"=w402:path)  [unwired: 2 in, 8 out]
            n258 = call <vilib>:"Open Config Data.vi"("configuration file path"=w402) -> ("refnum"=w400:T20)  [unwired: 8 in, 2 out]
          }
          frame True {
            n259 = property on="Camera Settings" class="Clust (strict)"("Visible"=TRUE) -> ()  [unwired: 2 in, 2 out]
          }
        }
      }
      event "Camera Settings": Value Change {
        # "Update summary string when any elements of DB camera change"
        n260 = event-data() -> ("NewVal"=w432:T2)  [unwired: 1 in]
        n261 = Index Array(array=w428) -> (element=w427:cluster{string[]})  [unwired: 1 in]
        n262 = Unbundle(w432) -> ("Frame Rate"=w423:i32, "Compression"=w422:i32, "Size"=w425:u16)
        n263 = Unbundle(w427) -> (w426:string[])
        n264 = Index Array(array=w426, index=w425) -> (element=w424:string)
        n265 = Format Into String(format string="%s   %dfps   %d%%", w424, w423, w422) -> (resulting string=w429:string)  [unwired: 2 in, 1 out]
        n266 = Build Array(w429) -> (w430:string[])
        n267 = property on="DB Camera Config" class="Bool (strict)"("Strings [4]"=w430) -> ()  [unwired: 2 in, 2 out]
      }
      event "Motor.Enable": Value Change {
        # "When the test mode otor enable helper is set, update that\ntree row item's value"
        n268 = event-data() -> ("NewVal"=w439:bool)  [unwired: 1 in]
        n269 = Unbundle("Motor") -> ("Value"=w438:dbl)  [unwired: 1 out]
        n270 = Select(t=w438, s=w439, f=0.0) -> (s? t:f=w436:dbl)
        n271 = call <vilib>:"NT Write Number.vi"("Numeric"=w436, "Name"=w435) -> ()  [unwired: 9 in, 1 out]
      }
      event "Test Slider": Value Change {
        # "When the test mode slider helper is set, update that\ntree row item's value"
        n272 = event-data() -> ("NewVal"=w443:dbl)  [unwired: 1 in]
        n273 = call <vilib>:"NT Write Number.vi"("Numeric"=w443, "Name"=w444) -> ()  [unwired: 9 in, 1 out]
      }
      event "On/Off": Value Change {
        # "When the test mode on/off helper value is set, update that\ntree row item's value"
        n274 = event-data() -> ("NewVal"=w449:bool)  [unwired: 1 in]
        n275 = Boolean To (0,1)(Boolean=w449) -> (0, 1=w448:i16)
        n276 = call <vilib>:"NT Write Number.vi"("Numeric"=w448, "Name"=w447) -> ()  [unwired: 9 in, 1 out]
      }
      event "Rev/Fwd": Value Change {
        # "When the test mode helper value for relays is set, update that\ntree row item's value"
        n277 = event-data() -> ("NewVal.Forward"=w458:bool, "NewVal.Reverse"=w457:bool)  [unwired: 1 in]
        n278 = Boolean To (0,1)(Boolean=w458) -> (0, 1=w454:i16)
        n279 = Boolean To (0,1)(Boolean=w457) -> (0, 1=w456:i16)
        n280 = Negate(x=w456) -> (-x=w455:i16)
        n281 = Add(x=w454, y=w455) -> (x+y=w453:i16)
        n282 = call <vilib>:"NT Write Number.vi"("Numeric"=w453, "Name"=w452) -> ()  [unwired: 9 in, 1 out]
      }
      event "Test Ring": Value Change {
        # "When a test mode helper value is selected from the ring,\nset the tree item's variable to the string value"
        n283 = event-data() -> ("NewVal"=w463:u16)  [unwired: 1 in]
        n284 = property on="Test Ring" class="Ring (strict)"() -> ("Strings []"=w464:string[])  [unwired: 2 in, 2 out]
        n285 = Index Array(array=w464, index=w463) -> (element=w462:string)
        n286 = call <vilib>:"NT Write String.vi"("String"=w462, "Name"=w461) -> ()  [unwired: 9 in, 1 out]
      }
      event "Rec Mode": Value Change {
        # "Update globals for recording mode and path to read log from.\nClear when logging and let NetworkTables set path for vision to\nuse."
        n287 = event-data() -> ("NewVal"=w476:enum32{"Stop", "Record", "Playback"})  [unwired: 1 in]
        n288 = global write "WPI_DashboardLogging Global.vi" "Logging Filename"(path "") -> ()
        n289 = global write "WPI_DashboardLogging Global.vi" "Recording"(w476) -> ()
        n290 = case shown="\"Playback\"" w476 {
          tunnel: w475 -> [_ w478 w487]
          tunnel: [_ _ w486] -> w472
          tunnel: [_ _ w485] -> _
          tunnel: w470 -> [_ _ w483]
          tunnel: cluster{i32, i32} {-250, 170} -> [_ _ w482]
          tunnel: [_ _ T23 {"Image Size"=TRUE, "Image Type"=TRUE, "Pixel Value"=TRUE, "ROI Information"=TRUE, "Zoom Factor"=FALSE} ("Image Information Shown:All Elements")] -> w468
          tunnel: [_ _ TRUE ("Zoom Factor")] -> w467
          tunnel: w466 -> [_ _ w479]
          frame Default {
          }
          frame "Stop", "Record" {
            # "Place Window too"
            n291 = invoke class="VI" method="FP.Close"(reference=w478) -> (reference out=w477:refnum<vi>)  [unwired: 2 in, 2 out]
            n292 = invoke class="VI" method="Abort VI"(reference=w477) -> ()  [unwired: 2 in, 3 out]
          }
          frame "Playback" {
            n293 = call "Open Playback Panel.vi"("Offset"=w482, "DB VI Ref"=w483, "Playback in"=w487) -> ("Playback out"=w484:refnum<vi>)  [unwired: 8 in]
            n294 = register-events(w484, w479) -> (reference out=w486:refnum<event-registration>, error out=w485:errorcluster)  [unwired: 2 in]
          }
        }
        n295 = property on="Camera Image" class="ImageControl"("Image Information Shown"=w468, "Image Information Visible"=w467) -> ()  [unwired: 2 in, 2 out]
        n296 = call <vilib>:"WPI_DashboardNT Log FieldName Cache.vi"("Operation"=enum16{"Lookup/Add", "Index", "Clear"}."Clear") -> ()  [unwired: 8 in, 3 out]
      }
      event Panel Close {
        w489 = enum32{"Stop", "Record", "Playback"}."Stop" ("Rec Mode")
        # "Playback window has been closed, abort"
        n297 = event-data() -> ()  [unwired: 1 in, 4 out]
        n298 = local write "Rec Mode"(w489) -> ()
        n299 = global write "WPI_DashboardLogging Global.vi" "Recording"(w489) -> ()
      }
      event Panel Close {
        # "Abort playback window and ourself"
        n300 = event-data() -> ()  [unwired: 1 in, 4 out]
        n301 = invoke class="VI" method="FP.Close"(reference=w495) -> (reference out=w494:refnum<vi>)  [unwired: 2 in, 2 out]
        n302 = invoke class="VI" method="Abort VI"(reference=w494) -> (error out=w493:errorcluster)  [unwired: 2 in, 2 out]
        n303 = invoke class="VI" method="Abort VI"(error in=w493) -> ()  [unwired: 2 in, 3 out]
      }
      event User Event {
        n304 = event-data() -> ("IDs"=w503:cluster{"RPC field ID":u16, "Unique ID":u16}, "String"=w502:string)  [unwired: 1 in]
        n305 = Bundle("IDs"=w503, "String"=w502) -> (w501:T9)  [unwired: 1 in]
        n306 = call <vilib>:"Retrieve RPC Response.vi"("RPC Response"=w501) -> ("Output"=w498:string[][])  [unwired: 10 in]
        n307 = Build Array (concatenate)(w496, w498) -> (w497:string[][])
        n308 = local write "Command Params"(w497) -> ()
        n309 = local write "Cmd Status"("" ("Cmd Status")) -> ()
      }
      event "Vision": Value Change {
        # "Enable/Disable Compression slider.\nHW USB is hard-coded into the camera"
        n310 = event-data() -> ("NewVal"=w510:u16)  [unwired: 1 in]
        n311 = Equal?(x=w510, y=u32 2 ("milliseconds to wait")) -> (x = y?=w508:bool)
        n312 = Select(t=T24."Disabled and Grayed Out" ("Disabled"), s=w508, f=T24."Enabled" ("Disabled")) -> (s? t:f=w505:T24)
        n313 = property on="Compression" class="Slide (strict)"("DisabledEnum"=w505) -> ()  [unwired: 2 in, 2 out]
      }
      event "Tree": Double Click {
        n314 = event-data() -> ("PlatMods"=w515:T27, "Tag"=w514:string)  [unwired: 1 in]
        n315 = Unbundle(w515) -> ("Shift"=w513:bool)  [unwired: 4 out]
        n316 = Not(x=w513) -> (.not. x?=w512:bool)
        n317 = call <vilib>:"NT Update Persistence.vi"("Persistence"=w512, "Name"=w514) -> ()  [unwired: 9 in, 1 out]
      }
    }
  }
  n318 = while {
    tunnel: w48 -> [w519]
    i -> [w522]
    stop <- FALSE stop-if-true
    n319 = Wait (ms)(milliseconds to wait=u32 100) -> ()  [unwired: 1 out]
    n320 = case shown="\"Playback\"" "Rec Mode" {
      tunnel: w522 -> [_ _ w537]
      tunnel: [u32 2829099 ("Base Color") u32 11141120 ("Target Color") w526] -> w518
      frame "Stop", Default {
        # "Reset the color, extra updates don't cost much"
      }
      frame "Record" {
      }
      frame "Playback" {
        # "Playback"
        n321 = Quotient & Remainder(x=w537, y=u32 50 ("milliseconds to wait")) -> (x-y*floor(x/y)=w533:u32)  [unwired: 1 out]
        n322 = Divide(x=w533, y=u32 50 ("milliseconds to wait")) -> (x/y=w530:dbl)
        n323 = Multiply(x=6.283185307179586, y=w530) -> (x*y=w535:dbl)
        n324 = Sine(x=w535) -> (sin(x)=w534:dbl)
        n325 = Absolute Value(x=w534) -> (abs(x)=w527:dbl)
        n326 = call "Interpolate RGB Color.vi"("Proportion"=w527, "Target Color"=u32 30976, "Base Color"=u32 2829099) -> ("Result Color"=w526:u32)  [unwired: 8 in]
      }
    }
    n327 = property class="Pane"(reference=w519, "PaneColor"=w518) -> ()  [unwired: 1 in, 2 out]
  }
  n328 = local write "Dashboard Tab"(T1."Drive" ("Dashboard Tab")) -> ()
  n329 = property on="On/Off" class="Bool (strict)"("Visible"=w16) -> ()  [unwired: 2 in, 2 out]
  n330 = property on="Motor" class="Clust (strict)"("Visible"=w16) -> ()  [unwired: 2 in, 2 out]
  n331 = property on="Progress" class="Clust (strict)"("Visible"=w16) -> ()  [unwired: 2 in, 2 out]
  n332 = property on="Test Ring" class="Ring (strict)"("Visible"=w16) -> ()  [unwired: 2 in, 2 out]
  n333 = property on="Rev/Fwd" class="Clust (strict)"("Visible"=w16) -> ()  [unwired: 2 in, 2 out]
  n334 = property on="Camera Settings" class="Clust (strict)"("Visible"=w16) -> ()  [unwired: 2 in, 2 out]
  n335 = while {
    tunnel: u16 1741 ("timeout ms (25000)") -> [w539]
    stop <- FALSE stop-if-true
    n336 = TCP Create Listener(10:w539) -> (0:w538:errorcluster, 3:w540:refnum<k5>)  [unwired: 4 in, 1 out]
    n337 = case shown="No Error" w538 {
      selector: w538 -> [w542 _]
      tunnel: w540 -> [w543 _]
      frame No Error {
        n338 = while {
          tunnel: w543 -> [w546]
          tunnel: w542 -> [w545]
          stop <- FALSE stop-if-true
          n339 = TCP Wait On Listener(8:w545, 11:w546) -> (0:w547:errorcluster, 4:w548:refnum<k5>)  [unwired: 2 in, 3 out]
          n340 = local write "TCP"(w548) -> ()
          n341 = case shown="No Error" w547 {
            frame No Error {
            }
            frame Error {
              n342 = Wait (ms)(milliseconds to wait=u32 1000) -> ()  [unwired: 1 out]
            }
          }
        }
      }
      frame Error {
        n343 = Wait (ms)(milliseconds to wait=u32 1000) -> ()  [unwired: 1 out]
      }
    }
  }
  n344 = local write "DB Camera Config"(w16) -> ()
  n345 = local write "Command Params"(string[][] [] ("Command Params")) -> ()
  n346 = global write "WPI_DashboardLogging Global.vi" "Recording"(w42) -> ()
  n347 = local write "Command Selection"(u16 0 ("milliseconds to wait")) -> ()
  n348 = local write "Rec Mode"(w42) -> ()
